vi "Create Table and add all Cells V2A.vi"(0 "PDF Report IN":refnum<class "PDF Report Class.lvclass">, 5 "Row background color":T20={"color"=16777225, "at each"=0}, 7 "Table properties":T18={"Table position"=1, "SpacingBefore (points)"=12.0, "SpacingAfter (points)"=12.0} {"Table position" items=["LEFT", "CENTER", "RIGHT"]}, 9 "PDF Table":refnum<class "Pdfp Table Class.lvclass">, 11 "error in (no error)":errorcluster, 12 "Row  [ ]":T1) -> (4 "PDF Report OUT":refnum<class "PDF Report Class.lvclass">, 8 "PdfPTable":refnum<k24>, 15 "error out":errorcluster)   [LabVIEW 2019]
doc: "<B>ENGLISH</B>\nAppends a table to the PDF document.\n\n<B>FRANÇAIS</B>\nAjoute un tableau au document PDF.\n\nVersion 2.0\nDeveloped by Jean-Marc Simard\nCopyright © 2013, Exaprom Inc.\nAll rights reserved.\nLicense: BSD\n\nWith iTextSharp 4.1.6 (http://itextsharp.sourceforge.net)\nunder Mozilla Public License Version 1.1\n(http://www.mozilla.org/MPL/MPL-1.1.html)"
uses:
  <userlib>/Exaprom PDF/LV Class/PDF Report Class/PDF Report Class.lvclass
  <userlib>/Exaprom PDF/Controls/Table Controls/Row Back Ground color Datas.ctl
  <userlib>/Exaprom PDF/Controls/Table Controls/Table properties.ctl
  <userlib>/Exaprom PDF/Controls/Table Controls/Table position.ctl
  <userlib>/Exaprom PDF/LV Class/Pdfp Table Class/Pdfp Table Class.lvclass
  C:/Program Files/National Instruments/LabVIEW 2019/user.lib/Exaprom PDF/DLL/itextsharp.dll
  DLL/itextsharp.dll
  <userlib>/Exaprom PDF/Controls/Table Controls/Table Appearance and Font Row [ ].ctl
  <userlib>/Exaprom PDF/Controls/Table Controls/One Row Appearance.ctl
  <userlib>/Exaprom PDF/Controls/Table Controls/Row from to.ctl
  <userlib>/Exaprom PDF/Controls/Table Controls/Cell, Alignment, LS and Font - hide Vmerge.ctl
  <userlib>/Exaprom PDF/Controls/Table Controls/Cell Type, Alignment and LS.ctl
  <userlib>/Exaprom PDF/Controls/Table Controls/Cell Alignment 20px.ctl
  <userlib>/Exaprom PDF/Controls/Table Controls/Text vertical arrangement.ctl
  <userlib>/Exaprom PDF/Controls/Text Controls/Line spacing.ctl
  <userlib>/Exaprom PDF/Controls/Table Controls/Cell Appearance.ctl
  <userlib>/Exaprom PDF/Controls/Table Controls/Cell Border 20 px.ctl
  <userlib>/Exaprom PDF/Controls/Table Controls/Merge Horizontal.ctl
  <userlib>/Exaprom PDF/Controls/Table Controls/Merge Vertical.ctl
  <userlib>/Exaprom PDF/Controls/Font Controls/Font complete cluster.ctl
  <userlib>/Exaprom PDF/Controls/Font Controls/Font size.ctl
  <userlib>/Exaprom PDF/Controls/Font Controls/Font color.ctl
  <userlib>/Exaprom PDF/Controls/Font Controls/Type and encoding.ctl
  <userlib>/Exaprom PDF/Controls/Text Controls/Unicode/Type and run direction.ctl
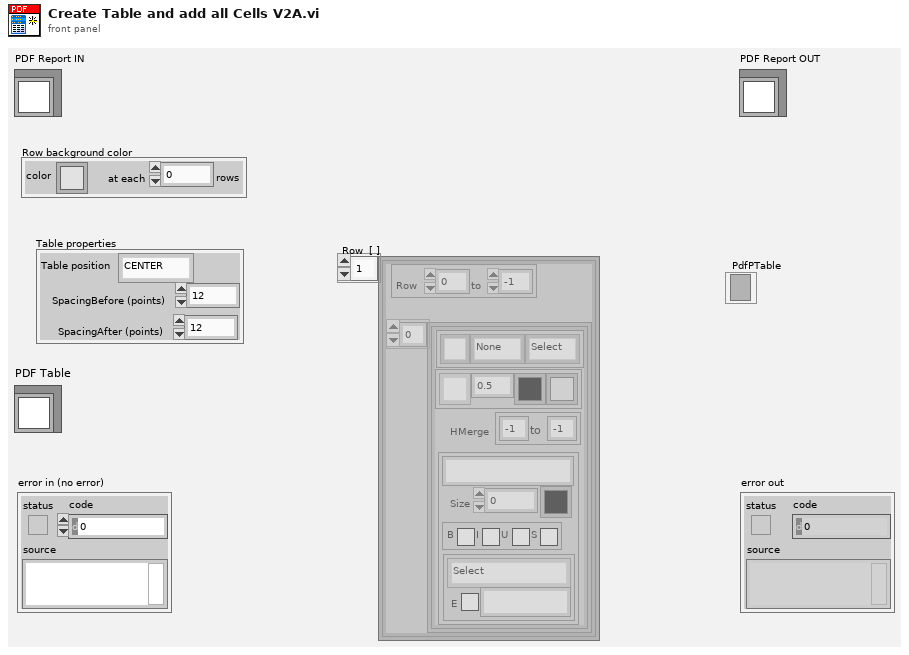
[diagram p1: front panel]
types:
  T1 = typedef "Table Appearance and Font Row [ ].ctl" = T2[]
  T2 = typedef "One Row Appearance.ctl" = cluster{"Row":T3, "Cell [ ]":T4[]}
  T3 = typedef "Row from to.ctl" = cluster{"From #":i16, "to #":i16}
  T4 = typedef "Cell, Alignment, LS and Font - hide Vmerge.ctl" = cluster{"Text":T5, "Cell Appearance":T9, "HMerge":T11, "VMerge":T12, "Font":T13}
  T5 = typedef "Cell Type, Alignment and LS.ctl" = cluster{"Cell Alignment":T6, "Text rotation":T7, "Line spacing":T8}
  T6 = typedef "Cell Alignment 20px.ctl" = u16
  T7 = typedef "Text vertical arrangement.ctl" = enum16{"None", "Clockwise", "Counterclockwise"}
  T8 = typedef "Line spacing.ctl" = enum16{"Select", "1.0", "1.5", "2.0"}
  T9 = typedef "Cell Appearance.ctl" = cluster{"Border":T10, "Thickness":sgl, "Color":u32, "BG":u32}
  T10 = typedef "Cell Border 20 px.ctl" = u16
  T11 = typedef "Merge Horizontal.ctl" = cluster{"From":i8, "to":i8}
  T12 = typedef "Merge Vertical.ctl" = cluster{"From":i8, "to":i8}
  T13 = typedef "Font complete cluster.ctl" = cluster{"Name":string, "Size":T14, "Color":T15, "Style":cluster{"Bold":bool, "Italic":bool, "Underline":bool, "Strikeout":bool}, "Type":T16}
  T14 = typedef "Font size.ctl" = sgl
  T15 = typedef "Font color.ctl" = u32
  T16 = typedef "Type and encoding.ctl" = cluster{"Type&direction":T17, "Embedded":bool, "Encoding":string}
  T17 = typedef "Type and run direction.ctl" = enum16{"Select", "ASCII", "UTF-16", "UTF-16 (default)", "UTF-16 (LTR)", "UTF-16 (RTL)"}
  T18 = typedef "Table properties.ctl" = cluster{"Table position":T19, "SpacingBefore (points)":sgl, "SpacingAfter (points)":sgl}
  T19 = typedef "Table position.ctl" = i32
  T20 = typedef "Row Back Ground color Datas.ctl" = cluster{"color":u32, "at each":i16}
  T21 = typedef "Image to Add [ ].ctl" = cluster{"Image name":string, "Path":path, "Scale":T22}[]
  T22 = typedef "Image Scale.ctl" = sgl
  T23 = typedef "Cell Cluster.ctl" = cluster{"Font Ref":refnum<k24>, "Close font ref":bool, "Type and run direction":T17, "Cell Alignment":T6, "Text rotation":T7, "Leading":T14, "PdfP Cell ref":refnum<k24>, "Colspan":i8}
  T24 = cluster{"Row":cluster{"#":i16, "to #":i16}, "Cell [ ]":T23[]}[]
  T25 = typedef "Image to Add refnum [ ].ctl" = cluster{"Image name":string, "InstanceImage":refnum<k24>}[]
  T26 = cluster{"Row":cluster{"#":i16, "to #":i16}, "Cell [ ]":T23[]}
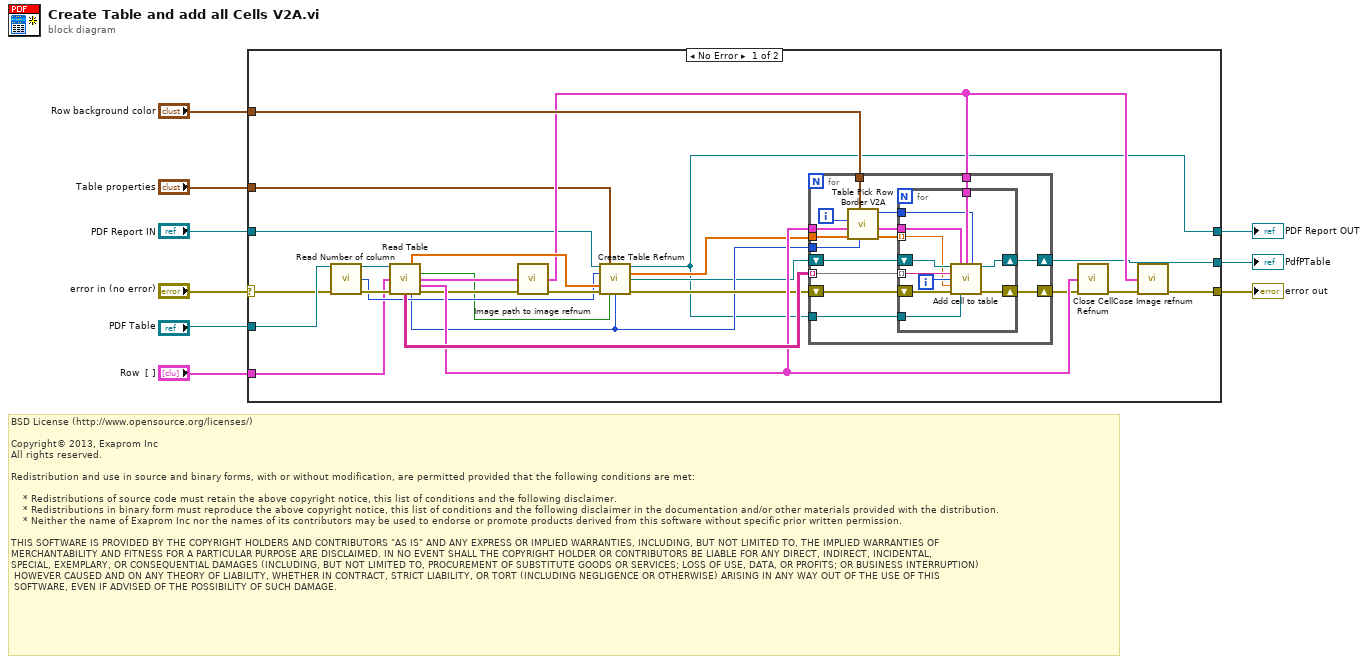
[diagram p0: block diagram]
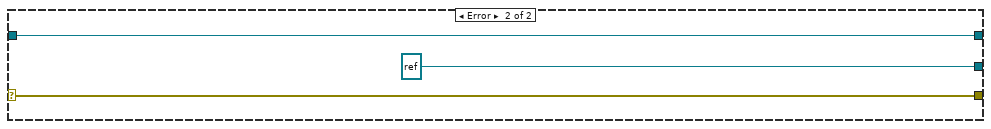
[diagram p2: hidden frame]
diagram:
  # "BSD License (http://www.opensource.org/licenses/)\n\nCopyright© 2013, Exaprom Inc\nAll rights reserved.\n\nRedistribution and use in source and binary forms, with or without modification, are permitted provided that the following conditions are met:\n\n    * Redistributions of source code must retain the above copyright notice, this list of conditions and the following disclaimer.\n    * Redistributions in binary form must reproduce the above copyright notice, this list of conditions and the following disclaimer in the documentation and/or other materials provided with the distribution.\n    * Neither the name of Exaprom Inc nor the names of its contributors may be used to endorse or promote products derived from this software without specific prior written permission.\n\nTHIS SOFTWARE IS PROVIDED BY THE COPYRIGHT HOLDERS AND CONTRIBUTORS \"AS IS\" AND ANY EXPRESS OR IMPLIED WARRANTIES, INCLUDING, BUT NOT LIMITED TO, THE IMPLIED WARRANTIES OF \nMERCHANTABILITY AND FITNESS FOR A PARTICULAR PURPOSE ARE DISCLAIMED. IN NO EVENT SHALL THE COPYRIGHT HOLDER OR CONTRIBUTORS BE LIABLE FOR ANY DIRECT, INDIRECT, INCIDENTAL,\nSPECIAL, EXEMPLARY, OR CONSEQUENTIAL DAMAGES (INCLUDING, BUT NOT LIMITED TO, PROCUREMENT OF SUBSTITUTE GOODS OR SERVICES; LOSS OF USE, DATA, OR PROFITS; OR BUSINESS INTERRUPTION)\n HOWEVER CAUSED AND ON ANY THEORY OF LIABILITY, WHETHER IN CONTRACT, STRICT LIABILITY, OR TORT (INCLUDING NEGLIGENCE OR OTHERWISE) ARISING IN ANY WAY OUT OF THE USE OF THIS\n SOFTWARE, EVEN IF ADVISED OF THE POSSIBILITY OF SUCH DAMAGE."
  n1 = case shown="No Error" "error in (no error)" {
    selector: "error in (no error)" -> [w19 w63]
    tunnel: "Table properties" -> [w24 _]
    tunnel: "PDF Report IN" -> [w18 w64]
    tunnel: "Row background color" -> [w35 _]
    tunnel: [w10 w64] -> w5
    tunnel: [w34 w63] -> w4
    tunnel: "PDF Table" -> [w22 _]
    tunnel: [w17 refnum<k24> refnum ("PdfP Table ref")] -> w2
    tunnel: "Row  [ ]" -> [w11 _]
    frame No Error {
      n2 = call <userlib>:"Read Number of column.vi"("PDF Table Class"=w22, "error in (no error)"=w19) -> ("PDF Table Class duplicate"=w21:refnum<class "Pdfp Table Class.lvclass">, "# columns"=w20:i32, "error duplicate"=w23:errorcluster)  [unwired: 11 in]
      n3 = call-dynamic "Read Table.vi"("PDF Table Class.lvclass in"=w21, "Row  [ ]"=w11, "error in (no error)"=w23) -> ("Table columnWidth [ ]"=w28:sgl[], "Repeat on each new page?"=w15:bool, "Image to Add [ ]"=w29:T21, "Row format with ref [ ]"=w31:T24, "Titles and Datas 2D [ ]"=w32:string[][], "HeaderRows"=w14:u16, "error out"=w26:errorcluster)  [unwired: 4 in, 2 out]
      n4 = call <userlib>:"Image path to image refnum.vi"("Image to Add [ ]"=w29, "error in (no error)"=w26) -> ("Image to Add refnum [ ]"=w27:T25, "error out"=w25:errorcluster)  [unwired: 12 out]
      n5 = call <userlib>:"Create Table Refnum.vi"("PDF Report"=w18, "Table properties"=w24, "numColumns"=w20, "columnWidth [ ]"=w28, "error in (no error)"=w25, "Repeat on each new page?"=w15, "HeaderRows"=w14) -> ("PDF Report duplicate"=w10:refnum<class "PDF Report Class.lvclass">, "columnWidth (points)"=w13:sgl[], "PdfP Table ref"=w12:refnum<k24>, "error out"=w30:errorcluster)  [unwired: 5 in]
      n6 = for {
        shift-right: [w50] -> w17
        shift-left: w12 -> [w48]
        shift-right: [w49] -> w16
        shift-left: w30 -> [w47]
        tunnel: w32 -> [w46] mode=indexing
        tunnel: w27 -> [w45]
        tunnel: w31 -> [w41]
        tunnel: w35 -> [w40]
        tunnel: w13 -> [w39]
        tunnel: w14 -> [w37]
        tunnel: w10 -> [w36]
        i -> [w43]
        n7 = call <userlib>:"Table Pick Row Border V2A.vi"("# header rows"=w37, "Data Row Back Ground color"=w40, "columnWidth (points)"=w39, "Row format with ref [ ]"=w41, "i"=w43) -> ("columnWidth (points) out"=w38:sgl[], "Row format with ref"=w44:T26, "Background Color"=w42:u32)  [unwired: 1 in, 3 out]
        n8 = for {
          shift-right: [w61] -> w50
          shift-left: w48 -> [w59]
          shift-right: [w60] -> w49
          shift-left: w47 -> [w58]
          tunnel: w46 -> [w57] mode=indexing
          tunnel: w45 -> [w56]
          tunnel: w44 -> [w54]
          tunnel: w42 -> [w53]
          tunnel: w38 -> [w52] mode=indexing
          tunnel: w36 -> [w51]
          i -> [w55]
          n9 = call <userlib>:"Add cell to table.vi"("PdfP Table"=w59, "Row format with ref 2"=w54, "Image to Add [ ]"=w56, "Back Ground Color"=w53, "String"=w57, "i"=w55, "Column Width (points)"=w52, "error in (no error)"=w58, "PDF Report IN"=w51) -> ("PdfP Table duplicate"=w61:refnum<k24>, "error out"=w60:errorcluster)  [unwired: 5 out]
        }
      }
      n10 = call <userlib>:"Close Cell Refnum.vi"("References [ ]"=w31, "error in (no error)"=w16) -> ("error out"=w33:errorcluster)  [unwired: 1 in, 12 out]
      n11 = call <userlib>:"Cose Image refnum.vi"("Image to Add refnum [ ]"=w27, "error in (no error)"=w33) -> ("error out"=w34:errorcluster)  [unwired: 13 out]
    }
    frame Error {
    }
  }
  "error out" <- w4
  "PDF Report OUT" <- w5
  "PdfPTable" <- w2
